vi "Calculate_drilling_path.vi"(4 "calibration_pos":dbl[][](array[numeric]), 6 "Refractive index of the sample":dbl, 7 "Drilling type":i64, 8 "Large_C":bool, 9 "Z-bias in pixels":dbl, 10 "Drilling path":path, 11 "file path (dialog if empty)":path) -> (3 "depth":dbl)   [LabVIEW 2021]
uses:
  <vilib>/Utility/file.llb/Read Delimited Spreadsheet (DBL).vi
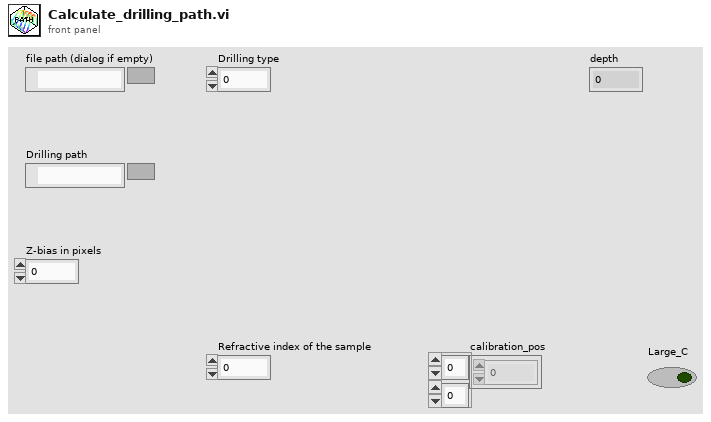
[diagram p1: front panel]
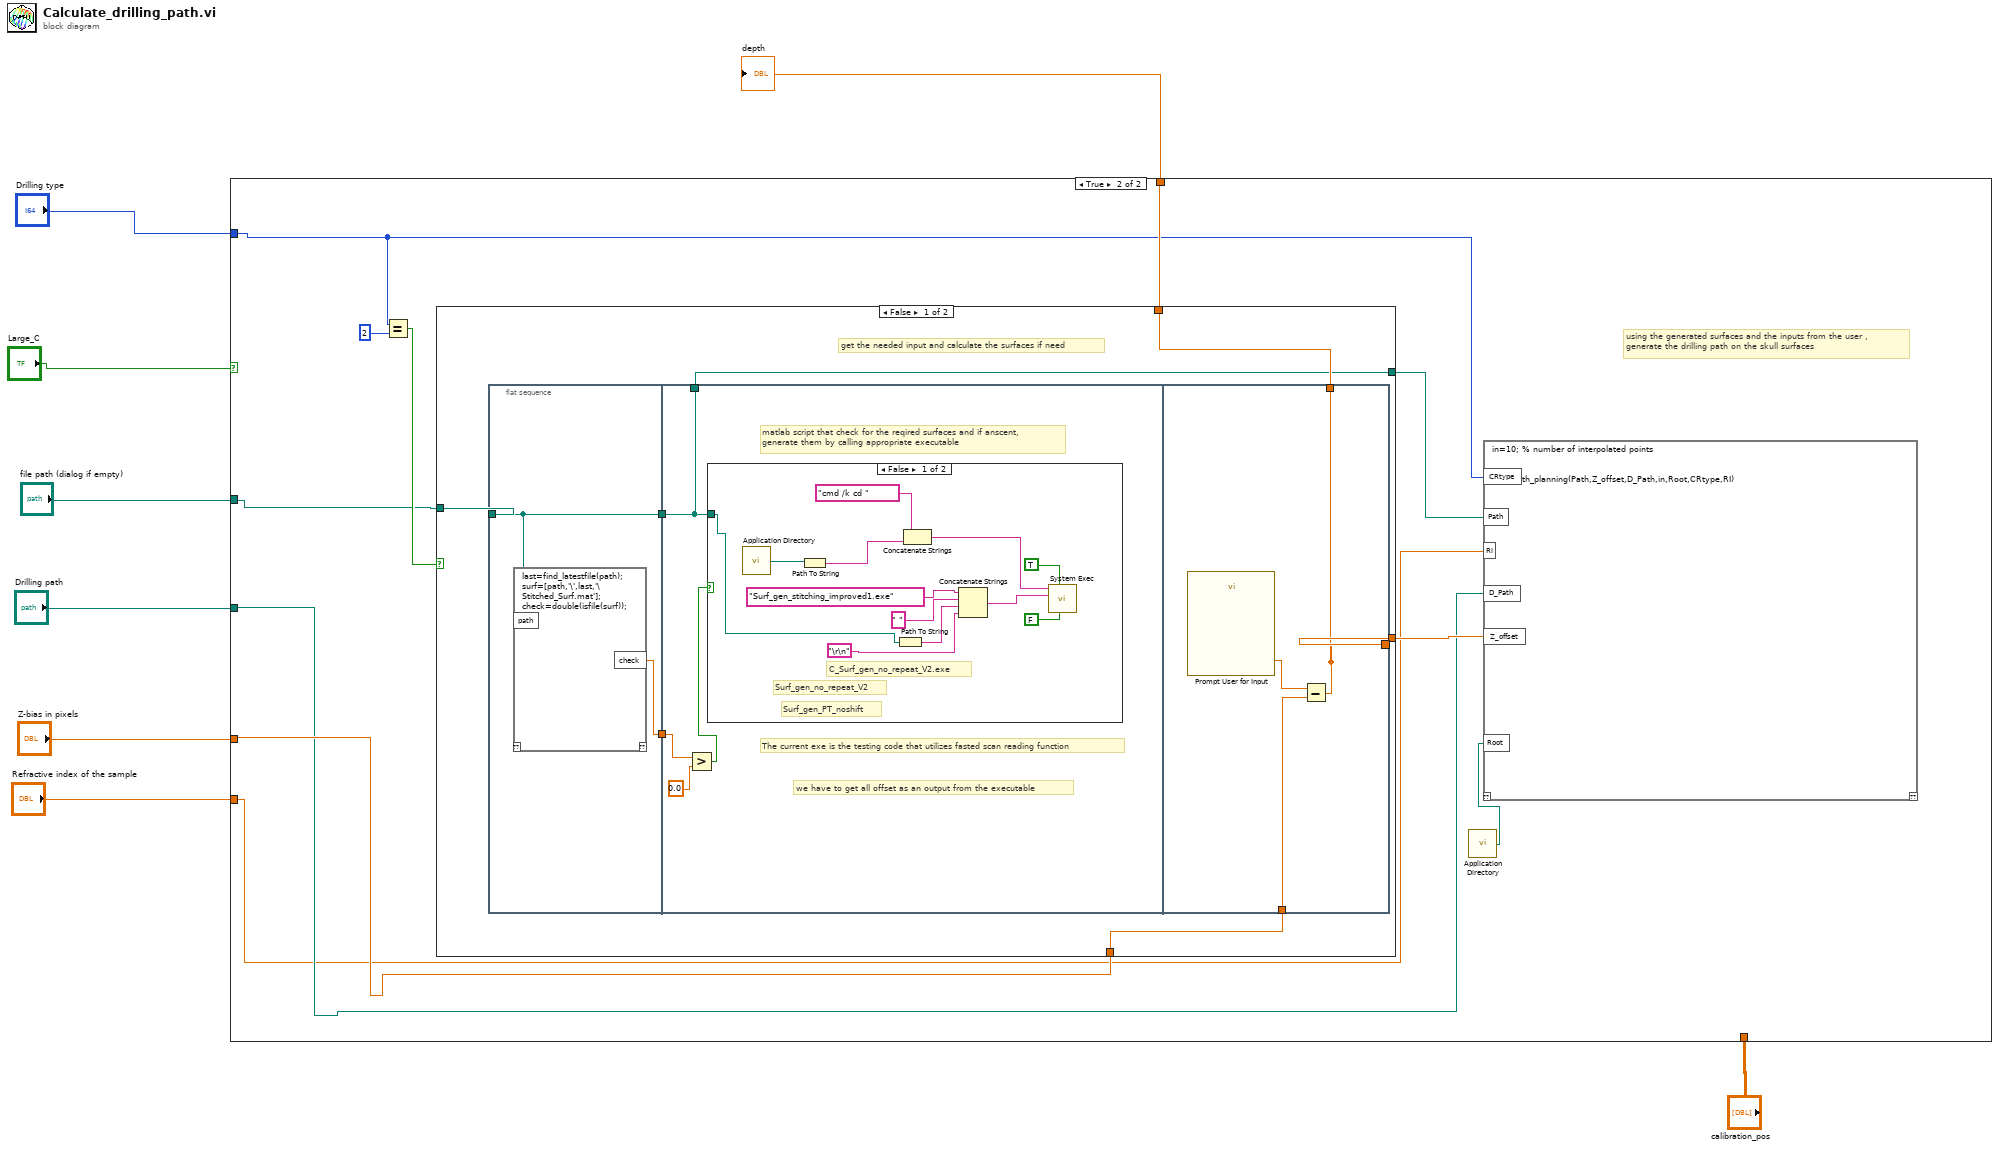
[diagram p0: block diagram]
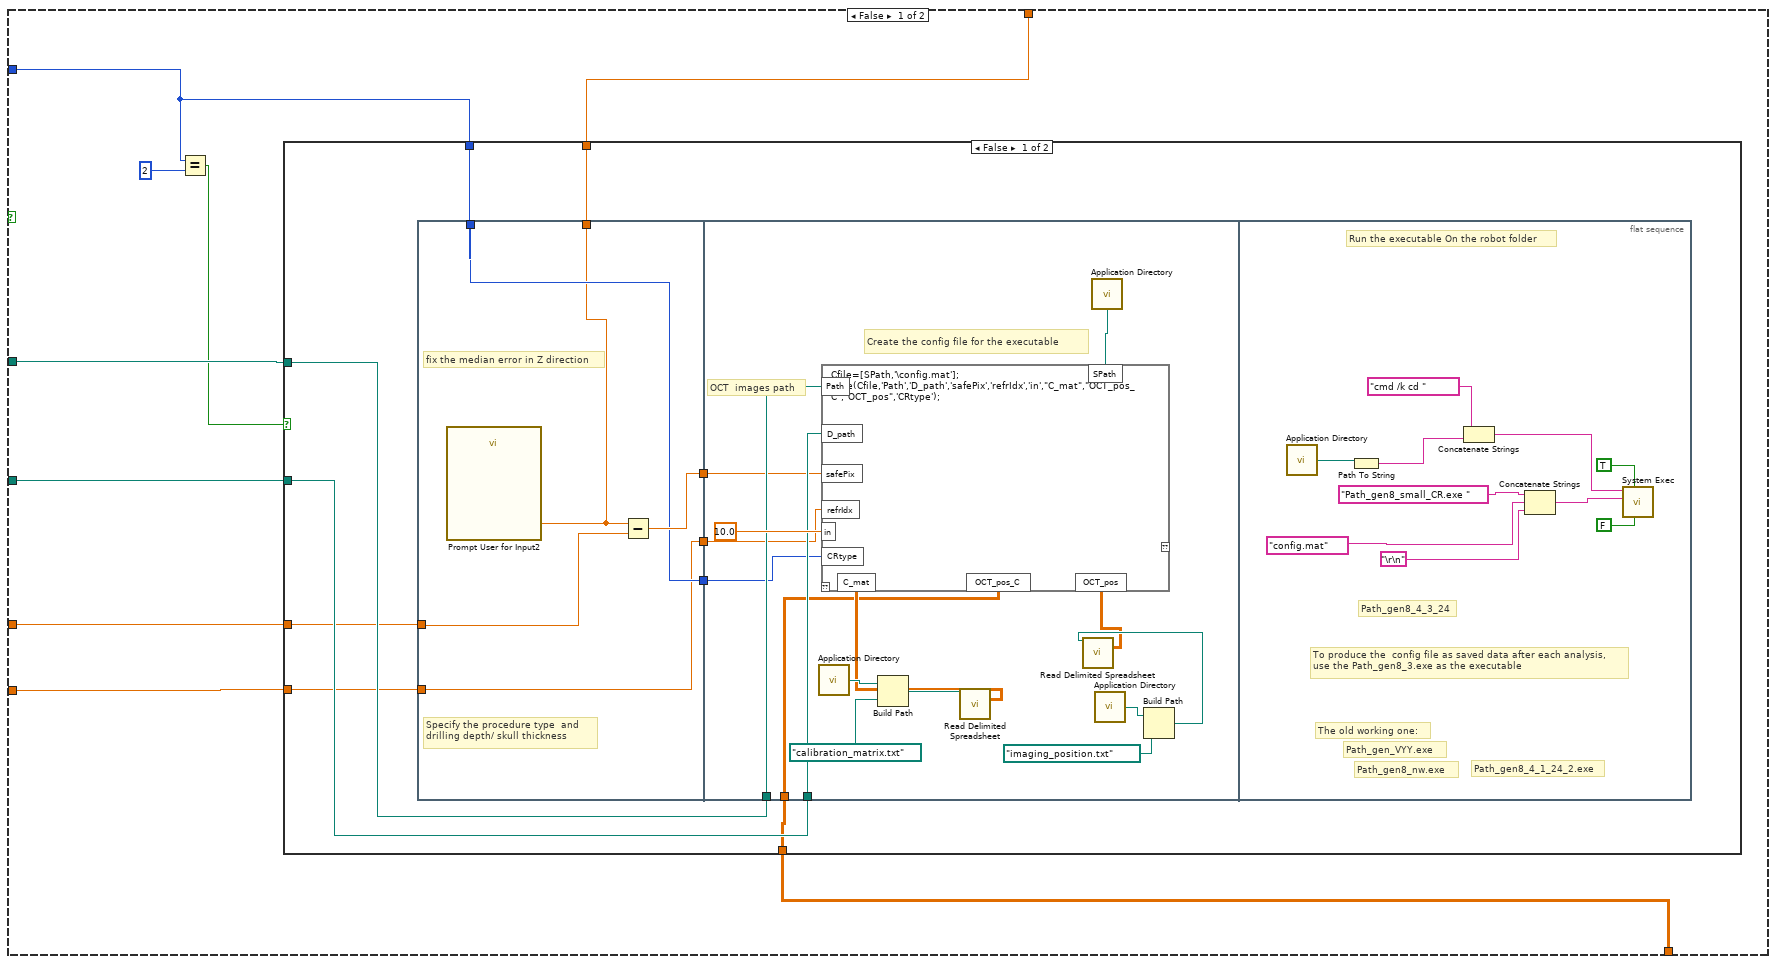
[diagram p2: hidden frame]
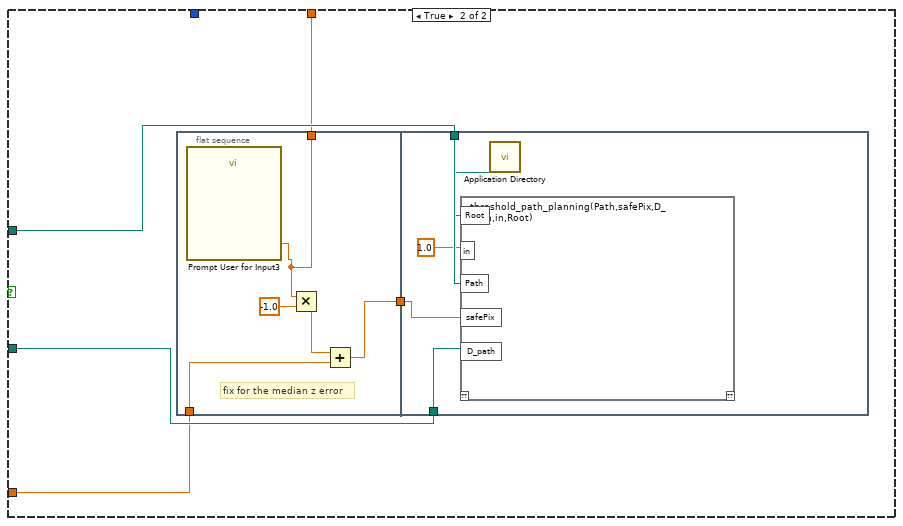
[diagram p3: hidden frame]
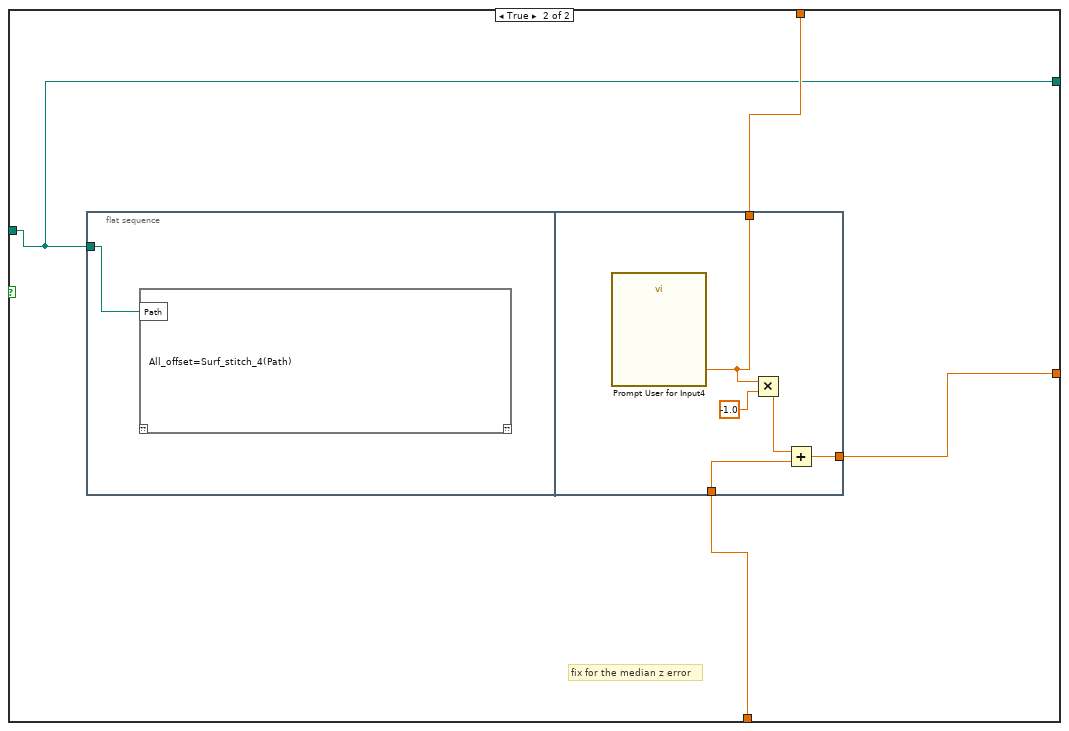
[diagram p5: hidden frame]
diagram:
  n1 = case shown="True" "Large_C" {
    tunnel: "calibration_pos" -> [w17 _]
    tunnel: "Refractive index of the sample" -> [w16 w76]
    tunnel: "Z-bias in pixels" -> [w15 w81]
    tunnel: "file path (dialog if empty)" -> [w14 w82]
    tunnel: [w13 w80] -> w4
    tunnel: "Drilling type" -> [w12 w75]
    tunnel: "Drilling path" -> [w11 w77]
    frame False {
      n2 = Equal?(x=w12, y=i64 2) -> (x = y?=w9:bool)
      n3 = case shown="False" w9 {
        tunnel: w11 -> [w24 w61]
        tunnel: w14 -> [w25 w62]
        tunnel: w12 -> [w27 _]
        tunnel: [w26 w60] -> w13
        tunnel: w15 -> [w21 w59]
        tunnel: w16 -> [w20 _]
        tunnel: w17 -> [w19 _]
        frame False {
          n4 = flat-sequence {
            tunnel: w27 -> [w31]
            tunnel: [w28] -> w26
            tunnel: [w32] -> w23
            tunnel: [w31] -> w22
            tunnel: w21 -> [w30]
            tunnel: w20 -> [w29]
            tunnel: [w29] -> w18
            tunnel: w25 -> [w46]
            tunnel: w24 -> [w45]
            tunnel: w23 -> [w43]
            tunnel: w22 -> [w42]
            tunnel: w19 -> [w33]
            tunnel: w18 -> [w44]
            frame #0 {
              # "fix the median error in Z direction"
              # "Specify the procedure type  and \ndrilling depth/ skull thickness"
              n5 = call "Prompt User for Input2"() -> ("thickness"=w28:dbl)  [unwired: 17 in, 2 out]
              n6 = Subtract(x=w28, y=w30) -> (x-y=w32:dbl)
            }
            frame #1 {
              # "OCT  images path"
              # "Create the config file for the executable"
              n7 = call <vilib>:"Application Directory.vi"() -> ("Application Directory"=w41:path)
              n8 = Build Path(base path=w41, name or relative path=path "calibration_matrix.txt" ("file path (dialog if empty)")) -> (appended path=w40:path)
              n9 = call-poly <vilib>:"Read Delimited Spreadsheet.vi"("file path (dialog if empty)"=w40) -> ("all rows"=w38:dbl[][])  [unwired: 9 in, 5 out]
              n10 = call <vilib>:"Application Directory.vi"() -> ("Application Directory"=w47:path)
              n11 = call <vilib>:"Application Directory.vi"() -> ("Application Directory"=w37:path)
              n12 = Build Path(base path=w37, name or relative path=path "imaging_position.txt" ("file path (dialog if empty)")) -> (appended path=w35:path)
              n13 = call-poly <vilib>:"Read Delimited Spreadsheet.vi"("file path (dialog if empty)"=w35) -> ("all rows"=w34:dbl[][])  [unwired: 9 in, 5 out]
              n14 = script code="Cfile=[SPath,'\\config.mat'];\nsave(Cfile,'Path','D_path','safePix','refrIdx','in',\"C_mat\",\"OCT_pos_C\",\"OCT_pos\",'CRtype');"("Path"=w46, "in"=10.0 ("Real"), "D_path"=w45, "safePix"=w43, "refrIdx"=w44, "C_mat"=w38, "OCT_pos"=w34, "OCT_pos_C"=w33, "CRtype"=w42, "SPath"=w47) -> ()  [unwired: 1 in, 1 out]
            }
            frame #2 {
              # "Path_gen8_4_3_24"
              # "Path_gen8_4_1_24_2.exe"
              # "Path_gen8_nw.exe"
              # "The old working one:"
              # "Path_gen_VYY.exe"
              # "To produce the  config file as saved data after each analysis,\nuse the Path_gen8_3.exe as the executable"
              # "Run the executable On the robot folder"
              n15 = call <vilib>:"Application Directory.vi"() -> ("Application Directory"=w51:path)
              n16 = Path To String(path=w51) -> (string=w50:string)
              n17 = Concatenate Strings("cmd /k cd " ("string"), w50) -> (w49:string)
              n18 = Concatenate Strings("Path_gen8_small_CR.exe " ("string"), "config.mat" ("string"), "\r\n") -> (w58:string)
              n19 = call <vilib>:"System Exec.vi"("run minimized? (F)"=FALSE, "wait until completion? (T)"=TRUE, "standard input"=w58, "command line"=w49) -> ()  [unwired: 4 in, 4 out]
            }
          }
        }
        frame True {
          n20 = flat-sequence {
            tunnel: [w66] -> w63
            tunnel: [w67] -> w60
            tunnel: w59 -> [w64]
            tunnel: w63 -> [w72]
            tunnel: w62 -> [w73]
            tunnel: w61 -> [w71]
            frame #0 {
              # "fix for the median z error"
              n21 = call "Prompt User for Input3"() -> ("depth"=w67:dbl)  [unwired: 17 in, 2 out]
              n22 = Multiply(x=w67, y=-1.0) -> (x*y=w65:dbl)
              n23 = Add(x=w65, y=w64) -> (x+y=w66:dbl)
            }
            frame #1 {
              n24 = call <vilib>:"Application Directory.vi"() -> ("Application Directory"=w69:path)
              n25 = script code="threshold_path_planning(Path,safePix,D_path,in,Root)"("in"=1.0 ("Real"), "Path"=w73, "safePix"=w72, "D_path"=w71, "Root"=w69) -> ()  [unwired: 1 in, 1 out]
            }
          }
        }
      }
    }
    frame True {
      # "using the generated surfaces and the inputs from the user ,\ngenerate the drilling path on the skull surfaces"
      n26 = Equal?(x=w75, y=i64 2) -> (x = y?=w83:bool)
      n27 = case shown="False" w83 {
        tunnel: w82 -> [w91 w113]
        tunnel: w81 -> [w90 w116]
        tunnel: [w89 w114] -> w80
        tunnel: [w88 w115] -> w79
        tunnel: [w87 w113] -> w78
        frame False {
          # "get the needed input and calculate the surfaces if need"
          n28 = flat-sequence {
            tunnel: w91 -> [w93]
            tunnel: [w93] -> w86
            tunnel: [w92] -> w85
            tunnel: [w97] -> w87
            tunnel: w86 -> [w97]
            tunnel: w85 -> [w95]
            tunnel: w90 -> [w112]
            tunnel: [w110] -> w89
            tunnel: [w110] -> w88
            frame #0 {
              n29 = script code="last=find_latestfile(path);\nsurf=[path,'\\',last,'\\Stitched_Surf.mat'];\ncheck=double(isfile(surf));"("path"=w93) -> ("check"=w92:dbl)  [unwired: 1 in, 1 out]
            }
            frame #1 {
              # "The current exe is the testing code that utilizes fasted scan reading function"
              # "we have to get all offset as an output from the executable"
              # "matlab script that check for the reqired surfaces and if anscent,\ngenerate them by calling appropriate executable"
              n30 = Greater?(x=w95, y=0.0) -> (0:w94:bool)
              n31 = case shown="False" w94 {
                tunnel: w97 -> [w100 _]
                frame False {
                  # "C_Surf_gen_no_repeat_V2.exe"
                  # "Surf_gen_PT_noshift"
                  # "Surf_gen_no_repeat_V2"
                  n32 = call <vilib>:"Application Directory.vi"() -> ("Application Directory"=w104:path)
                  n33 = Path To String(path=w104) -> (string=w103:string)
                  n34 = Path To String(path=w100) -> (string=w99:string)
                  n35 = Concatenate Strings("cmd /k cd " ("string"), w103) -> (w102:string)
                  n36 = Concatenate Strings("Surf_gen_stitching_improved1.exe" ("string"), " " ("string"), w99, "\r\n") -> (w109:string)
                  n37 = call <vilib>:"System Exec.vi"("run minimized? (F)"=FALSE, "wait until completion? (T)"=TRUE, "standard input"=w109, "command line"=w102) -> ()  [unwired: 4 in, 4 out]
                }
                frame True {
                }
              }
            }
            frame #2 {
              n38 = call "Prompt User for Input"() -> ("thickness"=w111:dbl)  [unwired: 17 in, 2 out]
              n39 = Subtract(x=w111, y=w112) -> (x-y=w110:dbl)
            }
          }
        }
        frame True {
          # "fix for the median z error"
          n40 = flat-sequence {
            tunnel: w113 -> [w117]
            tunnel: w116 -> [w118]
            tunnel: [w120] -> w115
            tunnel: [w119] -> w114
            frame #0 {
              n41 = script code="All_offset=Surf_stitch_4(Path)"("Path"=w117) -> ()  [unwired: 1 in, 1 out]
            }
            frame #1 {
              n42 = call "Prompt User for Input4"() -> ("depth"=w119:dbl)  [unwired: 17 in, 2 out]
              n43 = Multiply(x=w119, y=-1.0) -> (x*y=w122:dbl)
              n44 = Add(x=w122, y=w118) -> (x+y=w120:dbl)
            }
          }
        }
      }
      n45 = call <vilib>:"Application Directory.vi"() -> ("Application Directory"=w74:path)
      n46 = script code="in=10; % number of interpolated points\n\n\nLCR_path_planning(Path,Z_offset,D_Path,in,Root,CRtype,RI)"("Path"=w78, "RI"=w76, "D_Path"=w77, "Z_offset"=w79, "CRtype"=w75, "Root"=w74) -> ()  [unwired: 1 in, 1 out]
    }
  }
  "depth" <- w4
